vi "spectrograph.vi"() -> ()   [LabVIEW 2024]
uses:
  States.ctl
  <vilib>/Instr/_visa.llb/VISA Configure Serial Port (Instr).vi
panel:
  out "Array":dbl[](array[numeric])
  out "error out":errorcluster
  in  "stop":bool
  in  "Port":refnum<visa-resource-name>
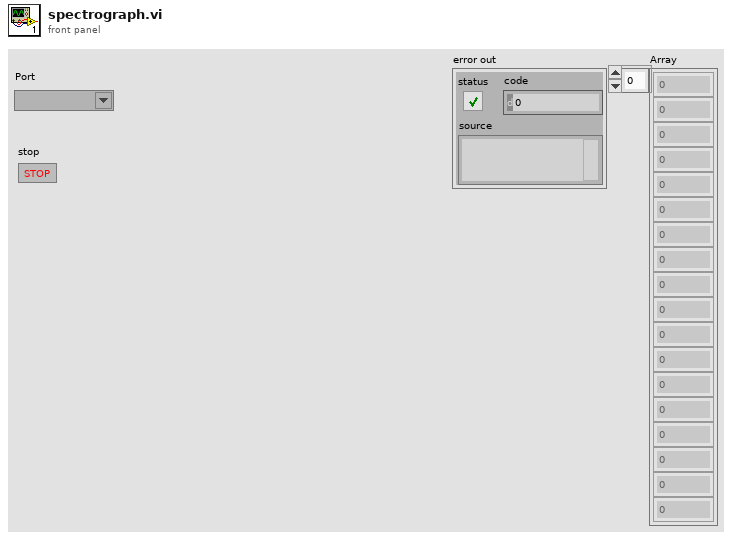
[diagram p1: front panel]
types:
  T1 = typedef "States.ctl" = enum16{"Initialize", "Loop", "Stop"}
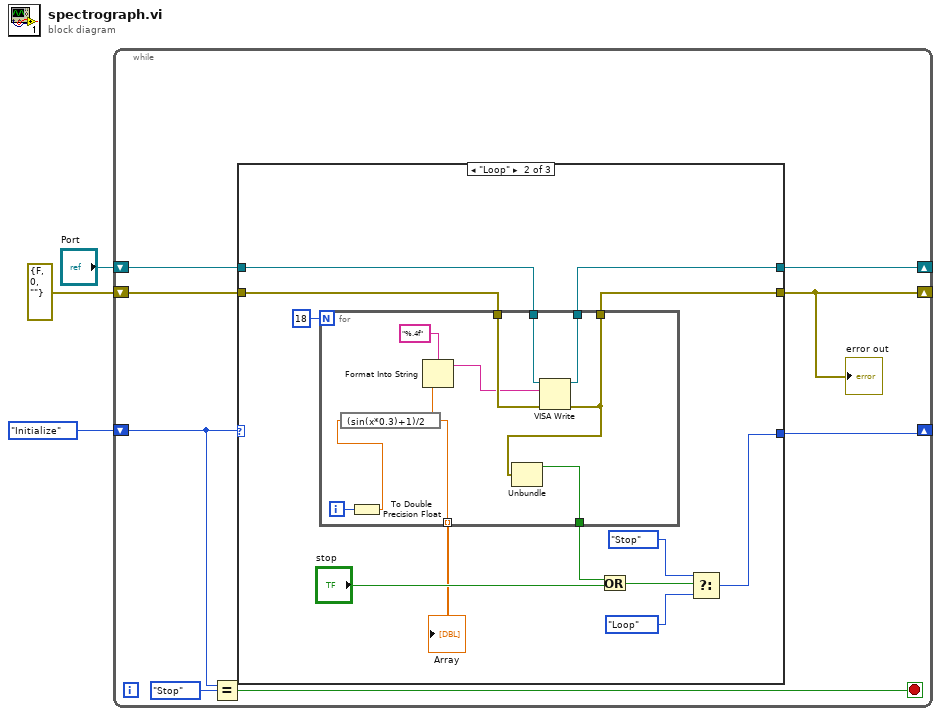
[diagram p0: block diagram]
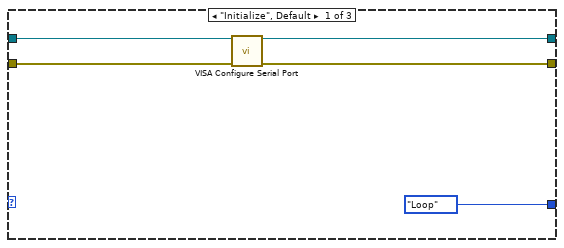
[diagram p2: hidden frame]
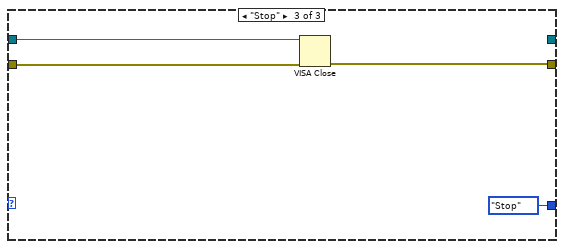
[diagram p3: hidden frame]
diagram:
  n1 = while {
    shift-right: [w9] -> _
    shift-left: "Port" -> [w10]
    shift-right: [w4] -> _
    shift-left: errorcluster {"status"=FALSE, "code"=0, "source"=""} ("error in (no error)") -> [w11]
    shift-right: [w7] -> _
    shift-left: States."Initialize" -> [w6]
    stop <- w8 stop-if-true
    n2 = Equal?(x=w6, y=States."Stop") -> (x = y?=w8:bool)
    n3 = case shown="\"Loop\"" w6 {
      tunnel: w10 -> [w16 w26 w42]
      tunnel: w11 -> [w15 w28 w41]
      tunnel: [w14 w25 _] -> w9
      tunnel: [w13 w27 w40] -> w4
      tunnel: [States."Loop" w21 States."Stop"] -> w7
      frame "Initialize", Default {
        n4 = call-poly "VISA Configure Serial Port"("VISA resource name"=w16, "error in (no error)"=w15) -> ("VISA resource name out"=w14:refnum<visa-resource-name>, "error out"=w13:errorcluster)  [unwired: 12 in]
      }
      frame "Loop" {
        n5 = for {
          N: 18 -> [_]
          tunnel: w28 -> [w36]
          tunnel: [w35] -> w27
          tunnel: w26 -> [w38]
          tunnel: [w37] -> w25
          tunnel: [w34] -> w18
          tunnel: [w30] -> w17 mode=indexing
          i -> [w29]
          n6 = To Double Precision Float(number=w29) -> (double precision float=w31:dbl)
          n7 = expression code="(sin(x*0.3)+1)/2"(w31) -> (w30:dbl)
          n8 = Format Into String(format string="%.4f", w30) -> (resulting string=w32:string)  [unwired: 2 in, 1 out]
          n9 = VISA Write(VISA resource name=w38, write buffer=w32, error in (no error)=w36) -> (VISA resource name out=w37:refnum<visa-resource-name>, error out=w35:errorcluster)  [unwired: 1 out]
          n10 = Unbundle(w35) -> ("status"=w34:bool)  [unwired: 2 out]
        }
        "Array" <- w17
        n11 = Or(x=w18, y="stop") -> (x .or. y?=w20:bool)
        n12 = Select(t=States."Stop", s=w20, f=States."Loop") -> (s? t:f=w21:T1)
      }
      frame "Stop" {
        n13 = VISA Close(VISA resource name=w42, error in (no error)=w41) -> (error out=w40:errorcluster)
      }
    }
    "error out" <- w4
  }
